vi "ASK调制与解调.vi"() -> ()   [LabVIEW 2013]
uses:
  <vilib>/measure/maspectr.llb/FFT Spectrum (Mag-Phase) for 1 Chan.vi
  <vilib>/Analysis/3filter.llb/Butterworth Filter (DBL).vi
  <vilib>/Analysis/NI_AALBase.lvlib
  <vilib>/measure/NI_MAPro.lvlib
panel:
  out "2ASK频谱图":cluster{"f0":dbl, "df":dbl, "magnitude":dbl[]}(graph)
  out "滤波后的波形":dbl[](graph)
  out "输出序列":u32[](array[numeric])
  out "滤波后的波形":dbl[](array[numeric]) caption="滤波后的X"
  in  "噪声标准差":dbl
  out "输入序列波形":dbl[](graph)
  out "2ASK波形":dbl[](graph)
  out "载波波形图":dbl[](graph)
  out "2ASK波形":dbl[](array[numeric])
  in  "相位输入":dbl
  in  "码速率RB":dbl
  in  "载波频率":dbl
  in  "采样率":dbl
  in  "采样点数N":dbl
  in  "输入序列":u32[](array[numeric]) format="%b"
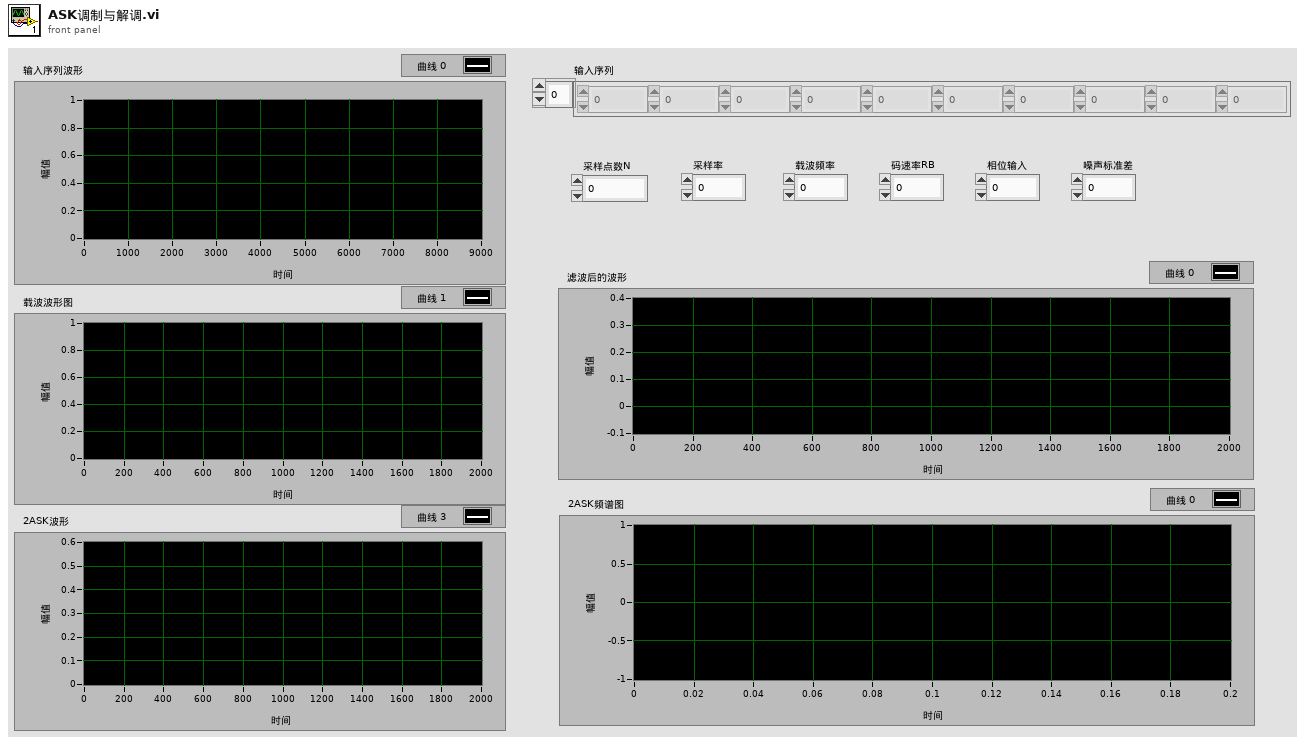
[diagram p1: front panel]
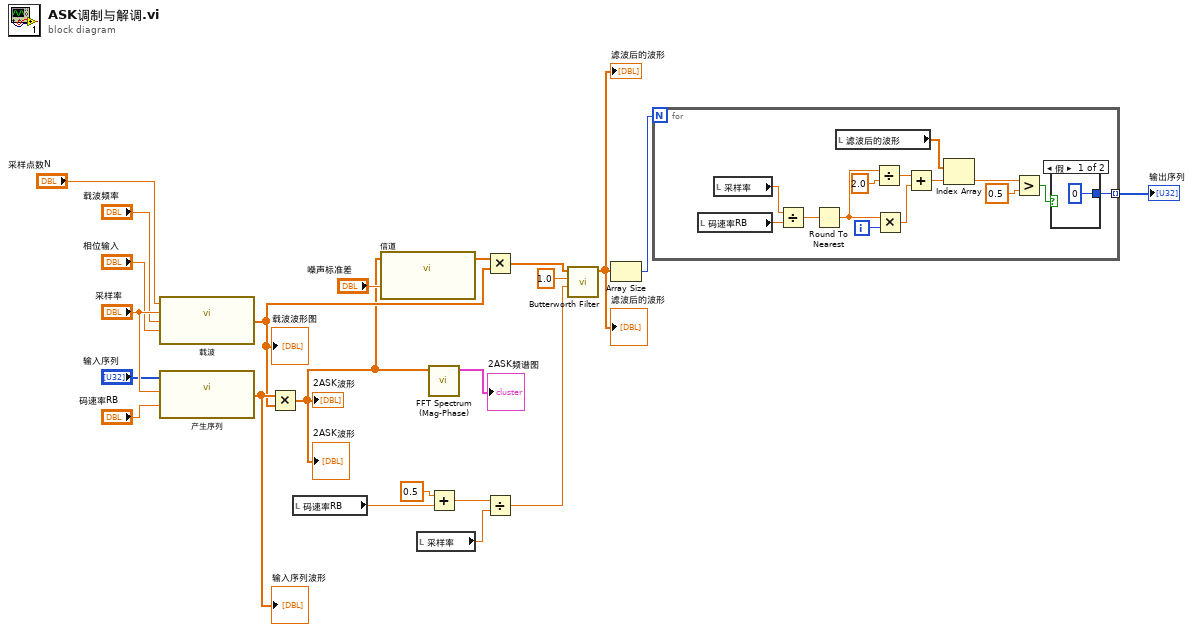
[diagram p0: block diagram]
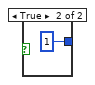
[diagram p2: hidden frame]
diagram:
  n1 = call "载波.vi"("相位输入"="相位输入", "载频"="载波频率", "采样率"="采样率", "采样点数"="采样点数N") -> ("载波信号波形"=w13:dbl[])
  "载波波形图" <- w13
  n2 = call "产生序列.vi"("码速率RB"="码速率RB", "采样率"="采样率", "输入序列"="输入序列") -> ("输入序列波形"=w16:dbl[])
  "输入序列波形" <- w16
  n3 = Multiply(x=w16, y=w13) -> (x*y=w3:dbl[])
  "2ASK波形" <- w3
  "2ASK波形" <- w3
  n4 = local read "码速率RB"() -> (w11:dbl)
  n5 = call "信道.vi"("噪声标准差"="噪声标准差", "调制信号"=w3) -> ("信道输出信号"=w14:dbl[])  [unwired: 1 out]
  n6 = local read "采样率"() -> (w9:dbl)
  n7 = call-poly <vilib>:"FFT Spectrum (Mag-Phase).vi"("time signal"=w3) -> ("magnitude"=→"2ASK频谱图":cluster{"f0":dbl, "df":dbl, "magnitude":dbl[]})  [unwired: 6 in, 4 out]
  n8 = Add(x=0.5, y=w11) -> (x+y=w8:dbl)
  n9 = Multiply(x=w14, y=w13) -> (x*y=w12:dbl[])
  n10 = Divide(x=w8, y=w9) -> (x/y=w7:dbl)
  n11 = call-poly <vilib>:"Butterworth Filter.vi"("high cutoff freq: fh"=w7, "sampling freq: fs"=1.0, "X"=w12) -> ("Filtered X"=w4:dbl[])  [unwired: 5 in, 1 out]
  "滤波后的波形" <- w4
  "滤波后的波形" <- w4
  n12 = Array Size(array=w4) -> (size(s)=w5:i32)
  n13 = for {
    N: w5 -> [_]
    tunnel: [w26] -> w1 mode=indexing
    i -> [w31]
    n14 = local read "码速率RB"() -> (w34:dbl)
    n15 = local read "采样率"() -> (w35:dbl)
    n16 = Divide(x=w35, y=w34) -> (x/y=w33:dbl)
    n17 = Round To Nearest(number=w33) -> (nearest integer value=w32:dbl)
    n18 = local read "滤波后的波形"() -> (w29:dbl[])
    n19 = Divide(x=w32, y=2.0) -> (x/y=w24:dbl)
    n20 = Multiply(x=w32, y=w31) -> (x*y=w25:dbl)
    n21 = Add(x=w24, y=w25) -> (x+y=w30:dbl)
    n22 = Index Array(array=w29, index=w30) -> (element=w23:dbl)
    n23 = Greater?(x=w23, y=0.5) -> (0:w27:bool)
    n24 = case shown="假" w27 {
      tunnel: [0 1] -> w26
      frame False {
      }
      frame True {
      }
    }
  }
  "输出序列" <- w1
